vi "UiDBCharts.vi"() -> ()   [LabVIEW 2011]
panel:
  out "XY Graph":cluster{timestamp, dbl}[](graph)
  in  "end":timestamp=timestamp(3427221599.999 s since 1904-01-01)
  in  "begin":timestamp=timestamp(3427135200 s since 1904-01-01)
  in  "sensor":T1(ring)
  in  "plant":enum16{"B2G1", "B2G2"}(ring)
  in  "load":bool
  in  "stop":bool
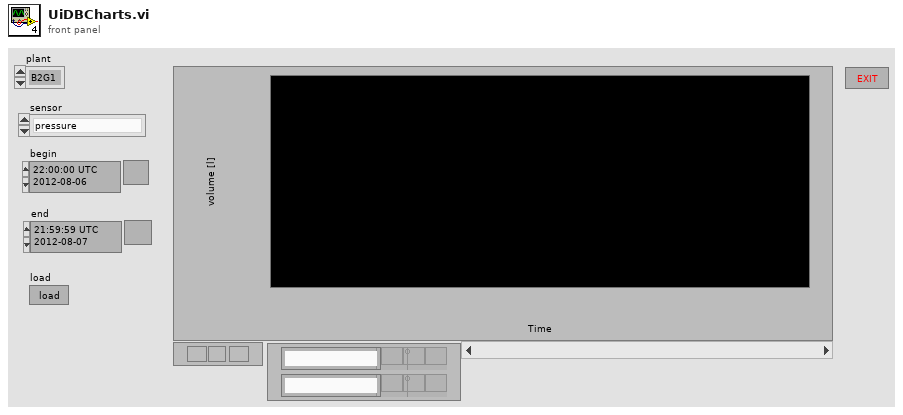
[diagram p1: front panel]
types:
  T1 = enum16{"pressure", "temperature 4", "temperature 5", "pH-value", "fill level 1", "fill level 2", "fill level 3"}
  T2 = enum32{"invalid app kind", "Development System", "Run Time System", "Student Edition", "Embedded LabVIEW", "Evaluation", "Custom"}
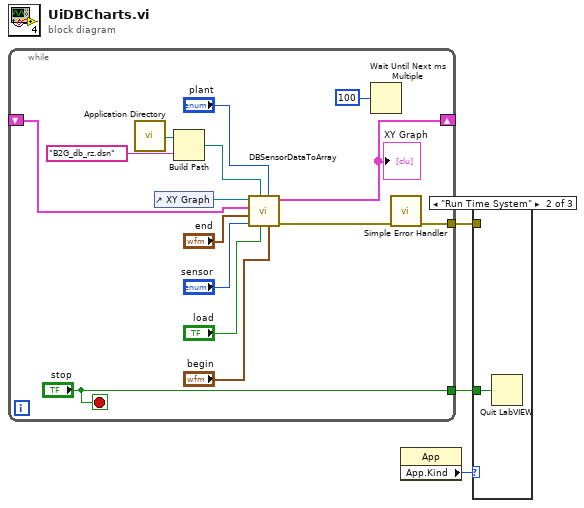
[diagram p0: block diagram]
diagram:
  n1 = while {
    shift-right: [w10] -> _
    shift-left: _ -> [w12]
    tunnel: ["stop"] -> w2
    tunnel: [w8] -> w1
    stop <- "stop" stop-if-true
    n2 = call <vilib>:"Application Directory.vi"() -> ("Application Directory"=w6:path)
    n3 = control-ref of="XY Graph"() -> (w4:refnum<vi>)
    n4 = Build Path(base path=w6, name or relative path="B2G_db_rz.dsn" ("Name of ini file 2")) -> (appended path=w5:path)
    n5 = call "DBSensorDataToArray.vi"("begin"="begin", "plant"="plant", "load"="load", "appended path"=w5, "sensor"="sensor", "end"="end", "shift reg out in"=w12, "XYGraph in"=w4) -> ("error out"=w11:errorcluster, "shift reg out"=w10:cluster{timestamp, dbl}[])  [unwired: 2 in]
    "XY Graph" <- w10
    n6 = Wait Until Next ms Multiple(millisecond multiple=u32 100) -> ()  [unwired: 1 out]
    n7 = call <vilib>:"Simple Error Handler.vi"("error in (no error)"=w11) -> ("error out"=w8:errorcluster)  [unwired: 4 in, 4 out]
  }
  n8 = property class="App"() -> ("App.Kind"=w3:T2)  [unwired: 2 in, 2 out]
  n9 = case shown="\"Run Time System\"" w3 {
    tunnel: w2 -> [_ w19 _]
    tunnel: w1 -> [_ _ _]
    frame "invalid app kind", Default {
    }
    frame "Run Time System" {
      n10 = Quit LabVIEW(quit? (T)=w19) -> ()
    }
    frame "Development System" {
    }
  }
